vi "GetWfrmSizes.vi"(8 "error in (no error)":errorcluster, 11 "FunctionBase in":refnum<class "FunctionBase.lvclass">) -> (0 "error out":errorcluster, 2 "WfrmSizes":i32[](array[numeric]), 3 "FunctionBase out":refnum<class "FunctionBase.lvclass">)   [LabVIEW 2018, in "Functions.lvlib" / "FunctionBase.lvclass"]
uses:
  FunctionBase.lvclass
  FunctionBase.lvclass/FunctionBase.ctl
  Accessors/Read Waveforms.vi
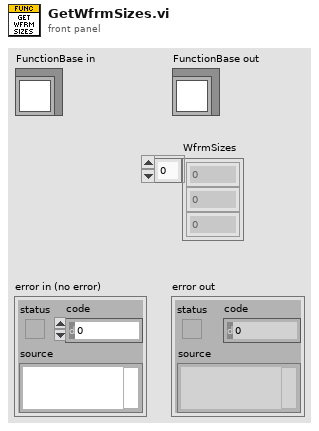
[diagram p1: front panel]
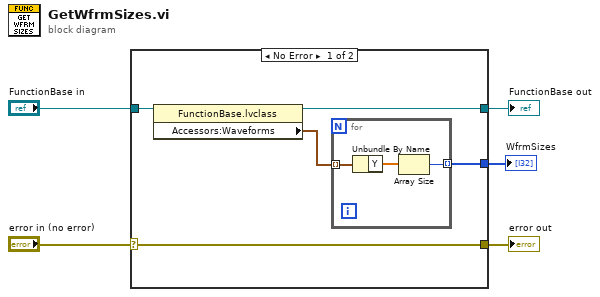
[diagram p0: block diagram]
diagram:
  n1 = case shown="No Error" "error in (no error)" {
    selector: "error in (no error)" -> [w9 w15]
    tunnel: [w9 w15] -> w4
    tunnel: [w8 w14] -> w2
    tunnel: "FunctionBase in" -> [w10 w14]
    tunnel: [w6 _] -> w1
    frame No Error {
      n2 = property class="FunctionBase.lvclass"(reference=w10) -> (reference out=w8:refnum<class "FunctionBase.lvclass">, "Accessors:Waveforms"=w7:waveform(dbl)[])  [unwired: 1 in, 1 out]
      n3 = for {
        tunnel: w7 -> [w13] mode=indexing
        tunnel: [w11] -> w6 mode=indexing
        n4 = Unbundle By Name(w13) -> ("Y"=w12:dbl[])
        n5 = Array Size(array=w12) -> (size(s)=w11:i32)
      }
    }
    frame Error {
    }
  }
  "error out" <- w4
  "FunctionBase out" <- w2
  "WfrmSizes" <- w1
